vi "Move t0 to the end.vi"(1 "waveform in":waveform(dbl)={"t0"=timestamp(0 s since 1904-01-01), "dt"=0.0, "Y"=[]}) -> (0 "waveform out":waveform(dbl))   [LabVIEW 2017]
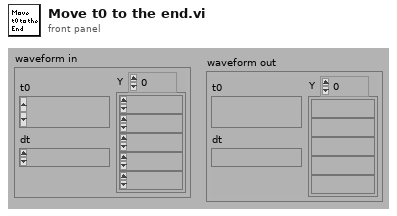
[diagram p1: front panel]
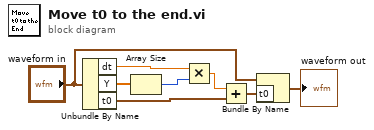
[diagram p0: block diagram]
diagram:
  n1 = Unbundle By Name("waveform in") -> ("dt"=w2:dbl, "Y"=w8:dbl[], "t0"=w6:timestamp)
  n2 = Array Size(array=w8) -> (size(s)=w1:i32)
  n3 = Multiply(x=w2, y=w1) -> (x*y=w7:dbl)
  n4 = Add(x=w7, y=w6) -> (x+y=w5:timestamp)
  n5 = Bundle By Name(cluster="waveform in", "t0"=w5) -> (→"waveform out":waveform(dbl))
